vi "IVIS FRET_Get Frame Time Stamp.vi"(8 "error in (no error)":errorcluster, 11 "File Path":path) -> (0 "error out":errorcluster, 3 "Time Stamp":i64)   [LabVIEW 2021]
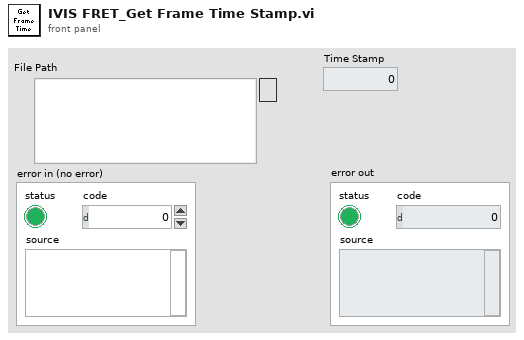
[diagram p1: front panel]
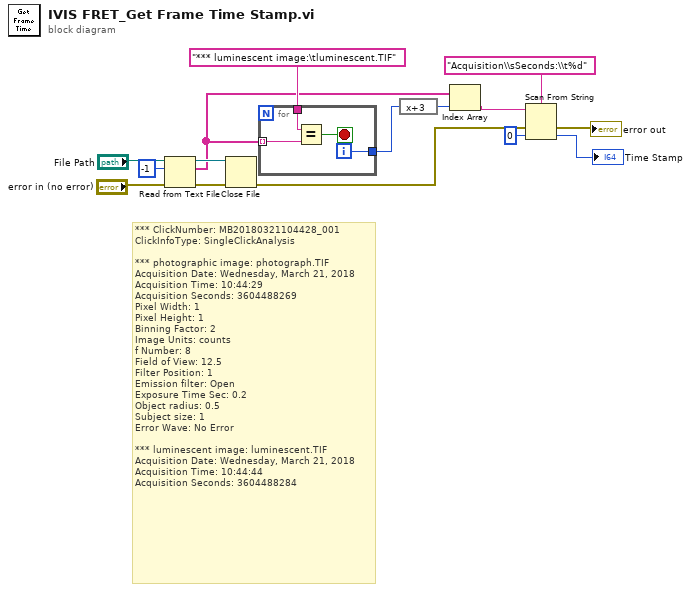
[diagram p0: block diagram]
diagram:
  # "*** ClickNumber:\tMB20180321104428_001\nClickInfoType:\tSingleClickAnalysis\n\n*** photographic image:\tphotograph.TIF\nAcquisition Date:\tWednesday, March 21, 2018\nAcquisition Time:\t10:44:29\nAcquisition Seconds:\t3604488269\nPixel Width:\t1\nPixel Height:\t1\nBinning Factor:\t2\nImage Units:\tcounts\nf Number:\t8\nField of View:\t12.5\nFilter Position:\t1\nEmission filter:\tOpen\nExposure Time Sec:\t0.2\nObject radius:\t0.5\nSubject size:\t1\nError Wave:\tNo Error\n\n*** luminescent image:\tluminescent.TIF\nAcquisition Date:\tWednesday, March 21, 2018\nAcquisition Time:\t10:44:44\nAcquisition Seconds:\t3604488284"
  n1 = Read from Text File(file (use dialog)="File Path", count=-1, error in="error in (no error)") -> (refnum out=w12:refnum<file>, text=w9:string[], error out=w11:errorcluster)  [unwired: 1 in, 1 out]
  n2 = Close File(refnum=w12, error in=w11) -> (error out=w4:errorcluster)  [unwired: 1 out]
  n3 = for {
    tunnel: w9 -> [w19] mode=indexing
    tunnel: "*** luminescent image:\tluminescent.TIF" ("x") -> [w18]
    tunnel: [w16] -> w8
    i -> [w16]
    stop <- w17 stop-if-true
    n4 = Equal?(x=w18, y=w19) -> (x = y?=w17:bool)
  }
  n5 = expression code="x+3"(w8) -> (w7:i32)
  n6 = Index Array(array=w9, index=w7) -> (element=w6:string)
  n7 = Scan From String(format string="Acquisition\\sSeconds:\\t%d", input string=w6, error in=w4, default 1=i64 0 ("default value 1")) -> (error out=→"error out":errorcluster, output 1=→"Time Stamp":i64)  [unwired: 1 in, 2 out]
